vi "ABB cleanup cool curve.vi"(9 "cool curve in":dbl[][](array[numeric])) -> (1 "Time":dbl[](array[numeric]), 2 "Cool curve out":dbl[][](array[numeric]), 3 "Resistance":dbl[](array[numeric]))   [LabVIEW 2017]
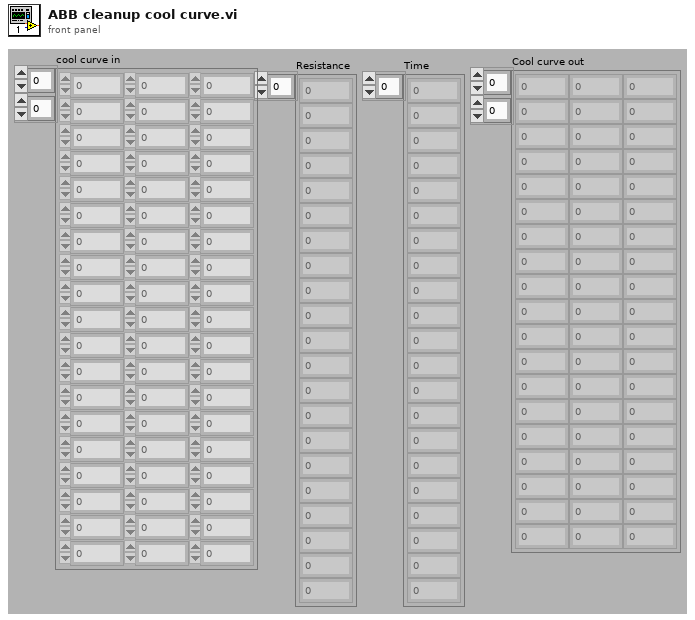
[diagram p1: front panel]
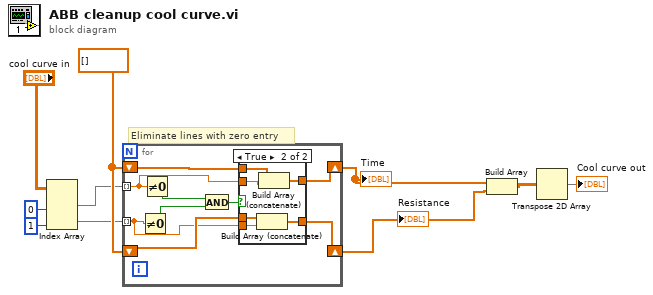
[diagram p0: block diagram]
diagram:
  w9 = dbl[] []
  # "Eliminate lines with zero entry"
  n1 = Index Array(array="cool curve in", index (col) #1=0 ("disabled index (col)"), index (col) #2=1 ("index (col)")) -> (element #1=w8:dbl[], element #2=w7:dbl[])  [unwired: 2 in]
  n2 = for {
    shift-right: [w16] -> w4
    shift-left: w9 -> [w17]
    shift-right: [w13] -> w3
    shift-left: w9 -> [w15]
    tunnel: w8 -> [w11] mode=indexing
    tunnel: w7 -> [w14] mode=indexing
    n3 = Not Equal To 0?(x=w14) -> (x != 0?=w19:bool)
    n4 = Not Equal To 0?(x=w11) -> (x != 0?=w12:bool)
    n5 = And(x=w12, y=w19) -> (x .and. y?=w18:bool)
    n6 = case shown="True" w18 {
      tunnel: w17 -> [w21 w27]
      tunnel: w11 -> [_ w26]
      tunnel: [w21 w25] -> w16
      tunnel: w15 -> [w20 w24]
      tunnel: w14 -> [_ w23]
      tunnel: [w20 w22] -> w13
      frame False {
      }
      frame True {
        n7 = Build Array (concatenate)(w24, w23) -> (w22:dbl[])
        n8 = Build Array (concatenate)(w27, w26) -> (w25:dbl[])
      }
    }
  }
  "Time" <- w4
  "Resistance" <- w3
  n9 = Build Array(w4, w3) -> (w2:dbl[][])
  n10 = Transpose 2D Array(2D array=w2) -> (transposed array=→"Cool curve out":dbl[][])
